vi "Autonomous.vi"   [LabVIEW 2016]
doc: "This VI starts when autonomous period begins, and will automatically be terminated when it ends. You can carry out timed or sensor driven operations directly to I/O or to subsystems without needing to return to the caller."
uses:
  <vilib>/Rock Robotics/Network Tables/NT Read String.vi
types:
  T1 = typedef "WPI_JoystickDevRef.ctl" = cluster{"Device":T2}
  T2 = typedef "WPI_JoystickDeviceEnum.ctl" = enum16{"USB 0", "USB 1", "USB 2", "USB 3", "USB 4", "USB 5"}
  T3 = typedef "Command Status Info.ctl" = cluster{"Name":string, "Status":T4, "notifier out":T5}
  T4 = typedef "Completion Status.ctl" = enum16{"Successful", "Aborted", "Incomplete"}
  T5 = typedef "Completion Notifier.ctl" = refnum<notifier>
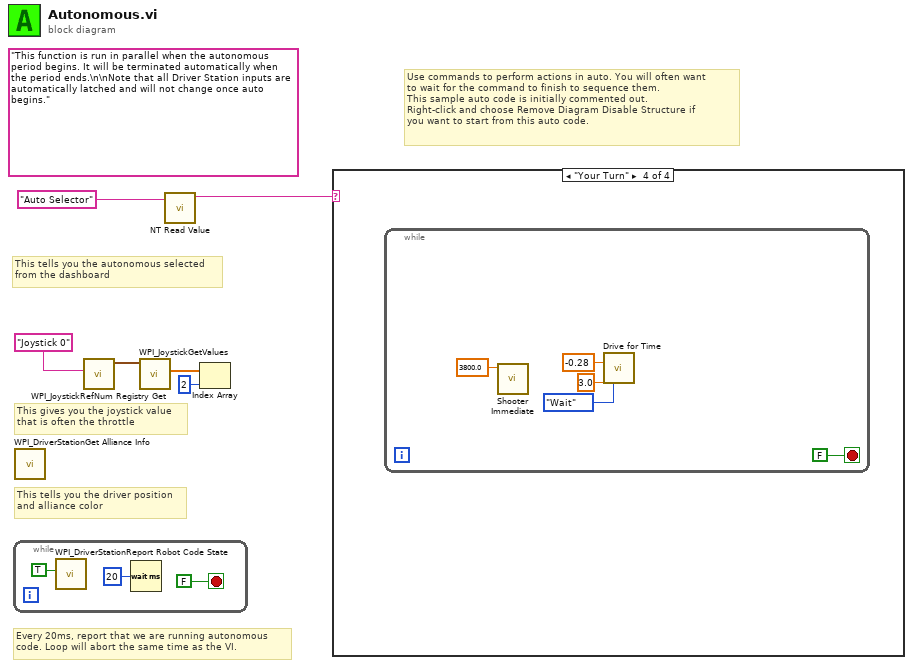
[diagram p0: block diagram]
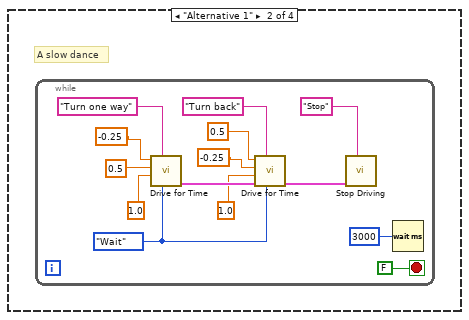
[diagram p3: hidden frame]
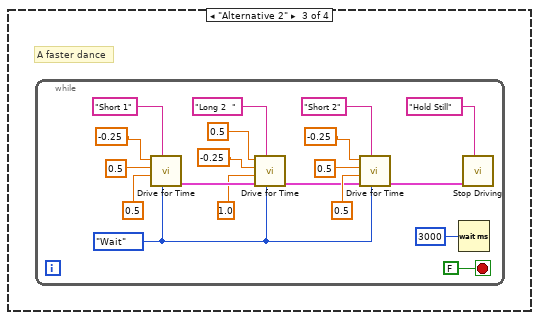
[diagram p4: hidden frame]
diagram:
  (unwired) "This function is run in parallel when the autonomous period begins. It will be terminated automatically when the period ends.\n\nNote that all Driver Station inputs are automatically latched and will not change once auto begins."
  # "This tells you the autonomous selected\nfrom the dashboard"
  # "Every 20ms, report that we are running autonomous\ncode. Loop will abort the same time as the VI."
  # "This gives you the joystick value\nthat is often the throttle"
  # "Use commands to perform actions in auto. You will often want\nto wait for the command to finish to sequence them.\nThis sample auto code is initially commented out. \nRight-click and choose Remove Diagram Disable Structure if\nyou want to start from this auto code."
  # "This tells you the driver position\nand alliance color"
  n1 = while {
    stop <- FALSE stop-if-true
    n2 = call <vilib>:"WPI_DriverStationReport Robot Code State.vi"("Autonomous"=TRUE) -> ()  [unwired: 10 in, 1 out]
    n3 = Wait (ms)(milliseconds to wait=u32 20) -> ()  [unwired: 1 out]
  }
  n4 = call <vilib>:"WPI_DriverStationGet Alliance Info.vi"() -> ()  [unwired: 12 out]
  n5 = call <vilib>:"WPI_JoystickRefNum Registry Get.vi"("refnum name"="Joystick 0") -> ("JoystickDevRef"=w5:T1)  [unwired: 1 in, 9 out]
  n6 = call <vilib>:"WPI_JoystickGetValues.vi"("JoystickDevRef"=w5) -> ("Axes"=w4:dbl[])  [unwired: 6 in, 4 out]
  n7 = call-poly <vilib>:"NT Read Value.vi"("Name"="Auto Selector") -> ("String"=w1:string)  [unwired: 9 in, 1 out]
  n8 = Index Array(array=w4, index=2) -> ()  [unwired: 1 out]
  n9 = case shown="\"Your Turn\"" w1 {
    frame Default {
      # "You can put your main auto here, or you can right-click on the case and make any\nother frame be the default case."
      # "This is the frame that will execute if no selection is made, or if it is not recognized"
    }
    frame "Alternative 1" {
      # "A slow dance"
      n10 = while {
        stop <- FALSE stop-if-true
        w14 = enum16{"Start", "Wait"}."Wait" ("Synchronication")
        n11 = call "Drive for Time.vi"("Synchronization"=w14, "Description"="Turn one way", "Seconds"=1.0 ("Delay (s)"), "Right Speed"=0.5 ("X axis value"), "Left Speed"=-0.25 ("X axis value")) -> ("Command Info Out"=w23:T3)  [unwired: 5 in, 1 out]
        n12 = call "Drive for Time.vi"("Synchronization"=w14, "Description"="Turn back", "Command Info In"=w23, "Seconds"=1.0 ("Delay (s)"), "Right Speed"=-0.25 ("X axis value"), "Left Speed"=0.5 ("X axis value")) -> ("Command Info Out"=w13:T3)  [unwired: 4 in, 1 out]
        n13 = call "Stop Driving.vi"("Description"="Stop", "Command Info In"=w13) -> ()  [unwired: 9 in, 1 out]
        n14 = Wait (ms)(milliseconds to wait=u32 3000 ("millisecond timer value")) -> ()  [unwired: 1 out]
      }
    }
    frame "Alternative 2" {
      # "A faster dance"
      n15 = while {
        stop <- FALSE stop-if-true
        w24 = enum16{"Start", "Wait"}."Wait" ("Synchronication")
        n16 = call "Drive for Time.vi"("Synchronization"=w24, "Description"="Short 1", "Seconds"=0.5 ("Delay (s)"), "Right Speed"=0.5 ("X axis value"), "Left Speed"=-0.25 ("X axis value")) -> ("Command Info Out"=w42:T3)  [unwired: 5 in, 1 out]
        n17 = call "Drive for Time.vi"("Synchronization"=w24, "Description"="Long 2  ", "Command Info In"=w42, "Seconds"=1.0 ("Delay (s)"), "Right Speed"=-0.25 ("X axis value"), "Left Speed"=0.5 ("X axis value")) -> ("Command Info Out"=w26:T3)  [unwired: 4 in, 1 out]
        n18 = call "Drive for Time.vi"("Synchronization"=w24, "Description"="Short 2", "Command Info In"=w26, "Seconds"=0.5 ("Delay (s)"), "Right Speed"=0.5 ("X axis value"), "Left Speed"=-0.25 ("X axis value")) -> ("Command Info Out"=w25:T3)  [unwired: 4 in, 1 out]
        n19 = Wait (ms)(milliseconds to wait=u32 3000 ("millisecond timer value")) -> ()  [unwired: 1 out]
        n20 = call "Stop Driving.vi"("Description"="Hold Still", "Command Info In"=w25) -> ()  [unwired: 9 in, 1 out]
      }
    }
    frame "Your Turn" {
      n21 = while {
        stop <- FALSE stop-if-true
        n22 = call "Shooter Immediate.vi"("Setpoint"=3800.0) -> ()  [unwired: 10 in, 1 out]
        n23 = call "Drive for Time.vi"("Y Speed"=-0.28, "Seconds"=3.0, "Synchronization"=enum16{"Start", "Wait"}."Wait") -> ()  [unwired: 11 in, 2 out]
      }
    }
  }
